vi "(SubVI) BM calculator.vi"(4 "BMy array in (nm)":dbl[](array[numeric]), 5 "y position array in (nm)":dbl[](array[numeric]) format="%0.2f", 6 "BMx array in (nm)":dbl[](array[numeric]), 7 "x position array in (nm)":dbl[](array[numeric]) format="%0.2f") -> (0 "BMy array appended (nm)":dbl[](array[numeric]), 2 "BMx array appended (nm)":dbl[](array[numeric]), 3 "Results":dbl[](array[numeric]))   [LabVIEW 2014]
uses:
  <vilib>/Analysis/baseanly.llb/Mean (DBL).vi
  <vilib>/Analysis/NI_AALBase.lvlib
panel:
  out "xy ratio":dbl
  out "updated BMy (nm)":dbl
  out "updated BMx (nm)":dbl
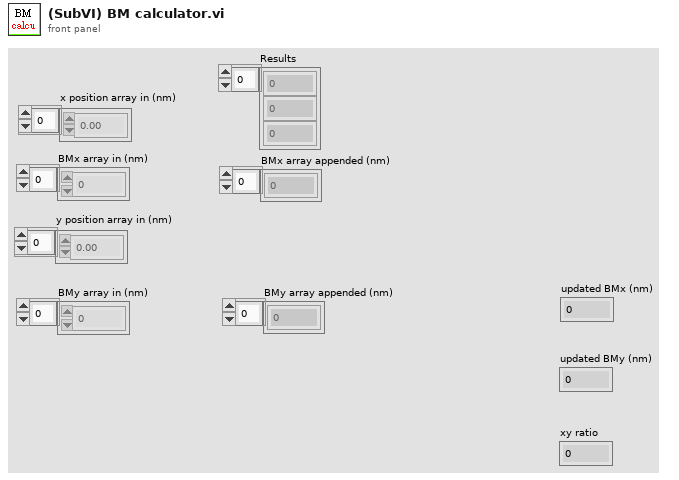
[diagram p1: front panel]
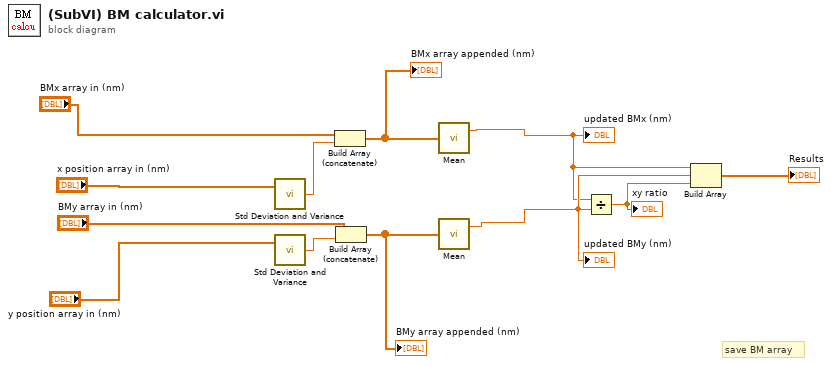
[diagram p0: block diagram]
diagram:
  # "save BM array"
  n1 = call <vilib>:"Std Deviation and Variance.vi"("X"="x position array in (nm)") -> ("standard deviation"=w1:dbl)  [unwired: 1 in, 2 out]
  n2 = call <vilib>:"Std Deviation and Variance.vi"("X"="y position array in (nm)") -> ("standard deviation"=w2:dbl)  [unwired: 1 in, 2 out]
  n3 = Build Array (concatenate)("BMx array in (nm)", w1) -> (w3:dbl[])
  "BMx array appended (nm)" <- w3
  n4 = Build Array (concatenate)("BMy array in (nm)", w2) -> (w4:dbl[])
  "BMy array appended (nm)" <- w4
  n5 = call-poly <vilib>:"Mean.vi"("X"=w3) -> ("mean"=w7:dbl)  [unwired: 1 out]
  "updated BMx (nm)" <- w7
  n6 = call-poly <vilib>:"Mean.vi"("X"=w4) -> ("mean"=w8:dbl)  [unwired: 1 out]
  "updated BMy (nm)" <- w8
  n7 = Divide(x=w7, y=w8) -> (x/y=w5:dbl)
  "xy ratio" <- w5
  n8 = Build Array(w7, w8, w5) -> (→"Results":dbl[])
